vi "From U64.vi"   [LabVIEW 2017]
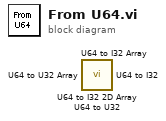
[diagram p0: block diagram]
diagram:
  n1 = call <vilib>:"U64 to I32 2D Array.vi"() -> ()  [unwired: 2 in, 2 out]
  n2 = call <vilib>:"U64 to I32 Array.vi"() -> ()  [unwired: 2 in, 2 out]
  n3 = call <vilib>:"U64 to U32 Array.vi"() -> ()  [unwired: 2 in, 2 out]
  n4 = call <vilib>:"U64 to I32.vi"() -> ()  [unwired: 2 in, 2 out]
  n5 = call <vilib>:"U64 to U32.vi"() -> ()  [unwired: 2 in, 2 out]
